vi "Nelson_Where_is_The_Whale.vi"(0 "Crosshair Bitmap":u32[][](array[colorbox]), 1 "Image In":T1, 2 "Image Copy":T1, 3 "error in":errorcluster, 4 "Color Based\nTracking?":bool=TRUE) -> (5 "Image":T1(plugin-control), 6 "Whale Position":cluster{"Y":dbl, "X":dbl}, 7 "error out":errorcluster)   [LabVIEW 2014]
uses:
  <vilib>/vision/Image Controls.llb/IMAQ Image.ctl
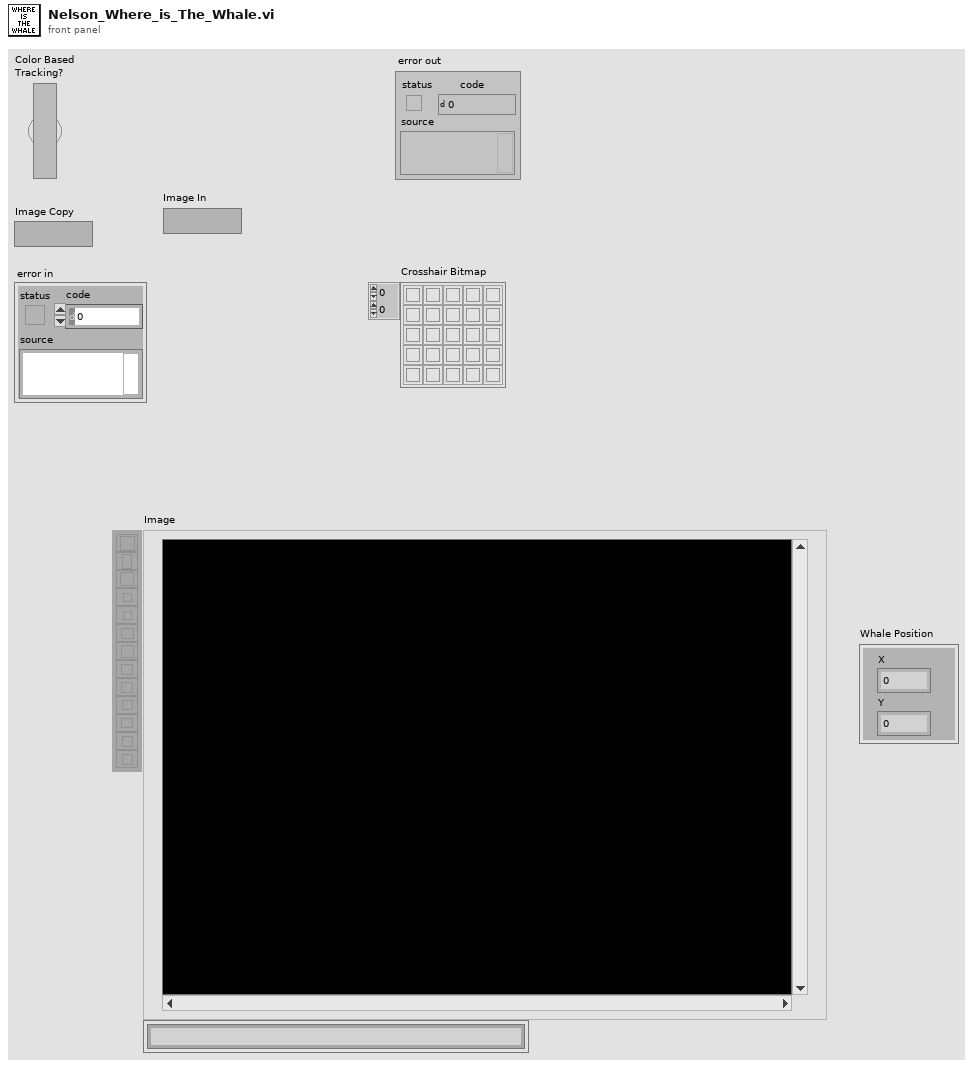
[diagram p1: front panel]
types:
  T1 = typedef "IMAQ Image.ctl" = refnum<image>
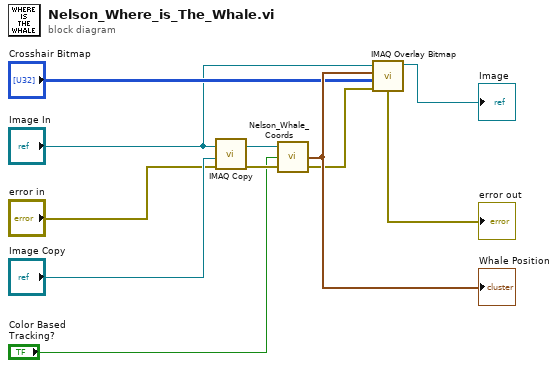
[diagram p0: block diagram]
diagram:
  n1 = call "IMAQ Copy"("error in (no error)"="error in", "Image Dst"="Image Copy", "Image Src"="Image In") -> ("error out"=w8:errorcluster, "Image Dst Out"=w7:T1)  [unwired: 3 in]
  n2 = call "Nelson_Whale_Coords.vi"("error in (no error)"=w8, "Color Based Tracking?"="Color Based\nTracking?", "Image"=w7) -> ("error out"=w10:errorcluster, "Position"=w11:cluster{"Y":dbl, "X":dbl})  [unwired: 1 out]
  "Whale Position" <- w11
  n3 = call "IMAQ Overlay Bitmap"("error in (no error)"=w10, "Bitmap"="Crosshair Bitmap", "Top Left Point"=w11, "Image"="Image In") -> ("error out"=→"error out":errorcluster, "Image Out"=→"Image":T1)  [unwired: 6 in]
